vi "System-Hidden-Settings-Host.vi"() -> ()   [LabVIEW 2016]
panel:
  in  "_Password":string caption="Password"
  in  "PiezoMinSwitch":sgl caption="[s]"
  in  "SolenoidMinSwitch":sgl caption="[s]"
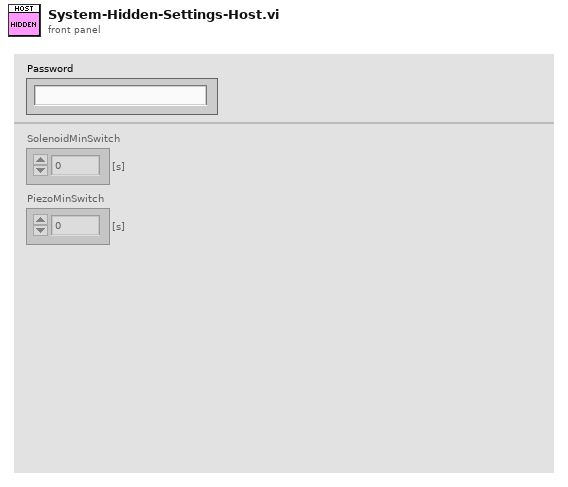
[diagram p1: front panel]
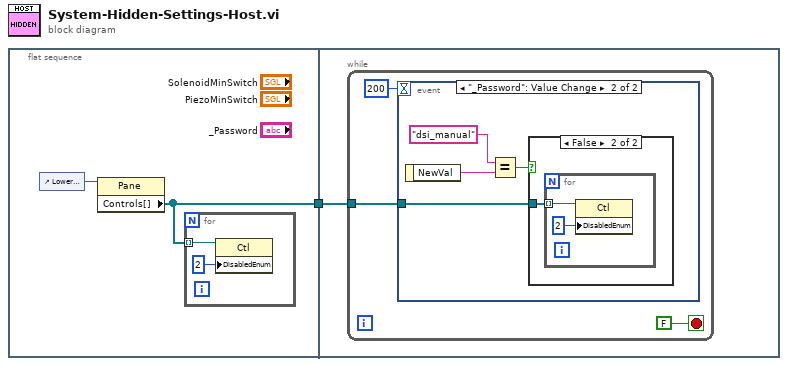
[diagram p0: block diagram]
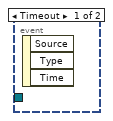
[diagram p2: hidden frame]
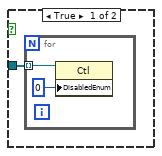
[diagram p3: hidden frame]
diagram:
  n1 = flat-sequence {
    tunnel: [w2] -> w1
    tunnel: w1 -> [w6]
    frame #0 {
      n2 = control-ref of="Lower Pane"() -> (w3:refnum<vi>)
      n3 = property class="Pane"(reference=w3) -> ("Controls[]"=w2:refnum<vi>[])  [unwired: 1 in, 2 out]
      n4 = for {
        tunnel: w2 -> [w5] mode=indexing
        n5 = property class="Ctl"(reference=w5, "DisabledEnum"=2) -> ()  [unwired: 1 in, 2 out]
      }
    }
    frame #1 {
      n6 = while {
        tunnel: w6 -> [w7]
        stop <- FALSE stop-if-true
        n7 = event shown="[1] \"_Password\": Value Change" {
          selector: _ -> [_ _]
          dyn-events: _ -> [_ _]
          timeout: 200 -> [_ _]
          tunnel: w7 -> [_ w11]
          event Timeout {
            n8 = event-data() -> ()  [unwired: 1 in, 3 out]
          }
          event "_Password": Value Change {
            n9 = event-data() -> ("NewVal"=w12:string)  [unwired: 1 in]
            n10 = Equal?(x="dsi_manual" ("y"), y=w12) -> (x = y?=w10:bool)
            n11 = case shown="False" w10 {
              tunnel: w11 -> [w14 w17]
              frame True {
                n12 = for {
                  tunnel: w14 -> [w15] mode=indexing
                  n13 = property class="Ctl"(reference=w15, "DisabledEnum"=0) -> ()  [unwired: 1 in, 2 out]
                }
              }
              frame False {
                n14 = for {
                  tunnel: w17 -> [w18] mode=indexing
                  n15 = property class="Ctl"(reference=w18, "DisabledEnum"=2) -> ()  [unwired: 1 in, 2 out]
                }
              }
            }
          }
        }
      }
    }
  }
